vi "Forebrain.vi"() -> ()   [LabVIEW 2011]
uses:
  Control 1.ctl
  MDF.ctl
  Behaviour.ctl
  Position.ctl
  WhereAmI.ctl
  ForebrainCmd.ctl
  <vilib>/userdefined/High Color/IMAQdx.ctl
  <vilib>/vision/Image Controls.llb/IMAQ Image.ctl
  OccGrid.ctl
  Behavior.vi
  <vilib>/vision/driver/NI_Vision_Acquisition_Software.lvlib
  <vilib>/vision/NI_Vision_Development_Module.lvlib
panel:
  in  "stop":bool
  out "Draw?":bool
  in  "Tab Control":T1(tab)
  in  "CompletedMDF":bool
  in  "ResetWaypoints":bool
  in  "Behaviour":T2
  out "No. of Waypoints":i16
  out "Waypoint Index":i16
  in  "Speed":dbl(slide) scale=0.0..10.0
  out "Mission Definition":T3
  out "Mission Def File":T4[](array[typedef])
  out "Occupancy Grid 2":T5(plugin-control)
  out "Behavior":string
  in  "Camera Name":T6
  out "Occupancy Grid":T5(plugin-control)
  out "x":sgl[](array[numeric])
  out "y":sgl[](array[numeric])
  out "OccupancyGrid (Raw Data)":i8[][](array[numeric])
  out "Working":bool
  in  "stop 2":bool
  out "Dock 2":cluster{"x":sgl, "y":sgl}
  out "Bouy 1":cluster{"x":sgl, "y":sgl}
  out "Boat 2":T7
  out "Nothing":cluster{"x":sgl, "y":sgl}
  out "Working Image":T5(plugin-control)
  in  "Camera/File?":bool
  in  "Image file name":string="real pool targets rotated.bmp"
  out "Wall Position 1":T4
  out "FB Act Command":dbl[](graph)
  out "Image":T5(plugin-control)
  out "Buoy2":T8
  out "Buoy1":T8
  out "Dock":T8
  out "Real-Time MDF":T4[](array[typedef])
  out "Boat":T7
  out "Current State":i32
  out "AutoModeStop":bool
  out "Forebrain Command":T9
  out "Alive?":bool
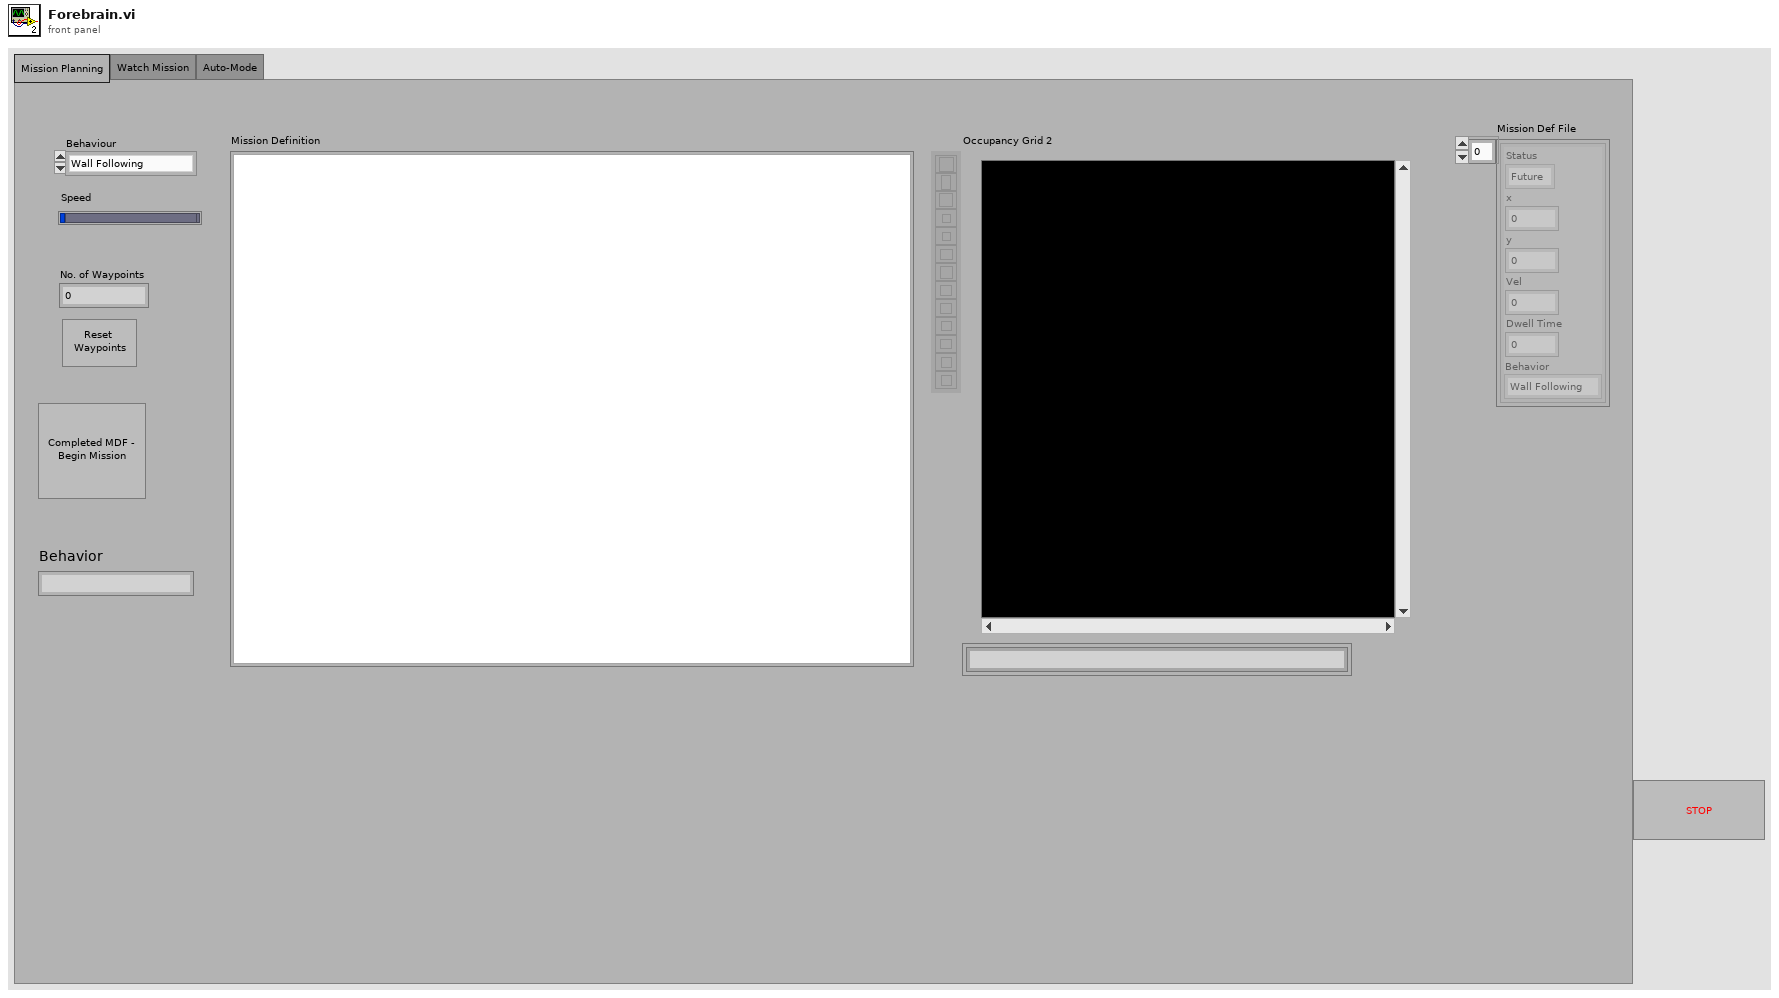
[diagram p1: front panel]
types:
  T1 = enum32{"Mission Planning", "Watch Mission", "Auto-Mode"}
  T2 = typedef "Behaviour.ctl" = enum16{"Wall Following", "Open Transit", "Find Barge", "Push Barge", "Go Home"}
  T3 = typedef "Control 1.ctl" = picture
  T4 = typedef "MDF.ctl" = cluster{"Status":enum16{"Past", "Current", "Future"}, "x":dbl, "y":dbl, "Vel":dbl, "Dwell Time":dbl, "Behavior":T2}
  T5 = typedef "IMAQ Image.ctl" = refnum<image>
  T6 = typedef "IMAQdx.ctl" = refnum<k21>
  T7 = typedef "WhereAmI.ctl" = cluster{"x":sgl, "y":sgl, "Boat\nHeading":sgl}
  T8 = typedef "Position.ctl" = cluster{"X":sgl, "Y":sgl}
  T9 = typedef "ForebrainCmd.ctl" = cluster{"Velocity":dbl, "Behaviour":T2}
  T10 = typedef "Image Type" = u32
  T11 = cluster{"Status":enum16{"Past", "Current", "Future"}, "x":dbl, "y":dbl, "Vel":dbl, "Dwell Time":dbl, "Behavior":T2}[]
  T12 = cluster{"Width":u16, "Style":enum32{"Solid", "Dash", "Dot", "DashDot", "DashDotDot"}}
  T13 = cluster{"Status":enum16{"Past", "Current", "Future"}, "x":dbl, "y":dbl, "Vel":dbl, "Dwell Time":dbl, "Behaviour":T2}
  T14 = typedef "OccGrid.ctl" = i16[][]
  T15 = typedef "LVMouseTypeDef.ctl" = cluster{"Mouse Position":cluster{"X":i32, "Y":i32}, "Mouse Modifiers":cluster{"Button Down":bool, "Shift Mod":bool, "Menu Mod":bool, "Option Mod":bool}}
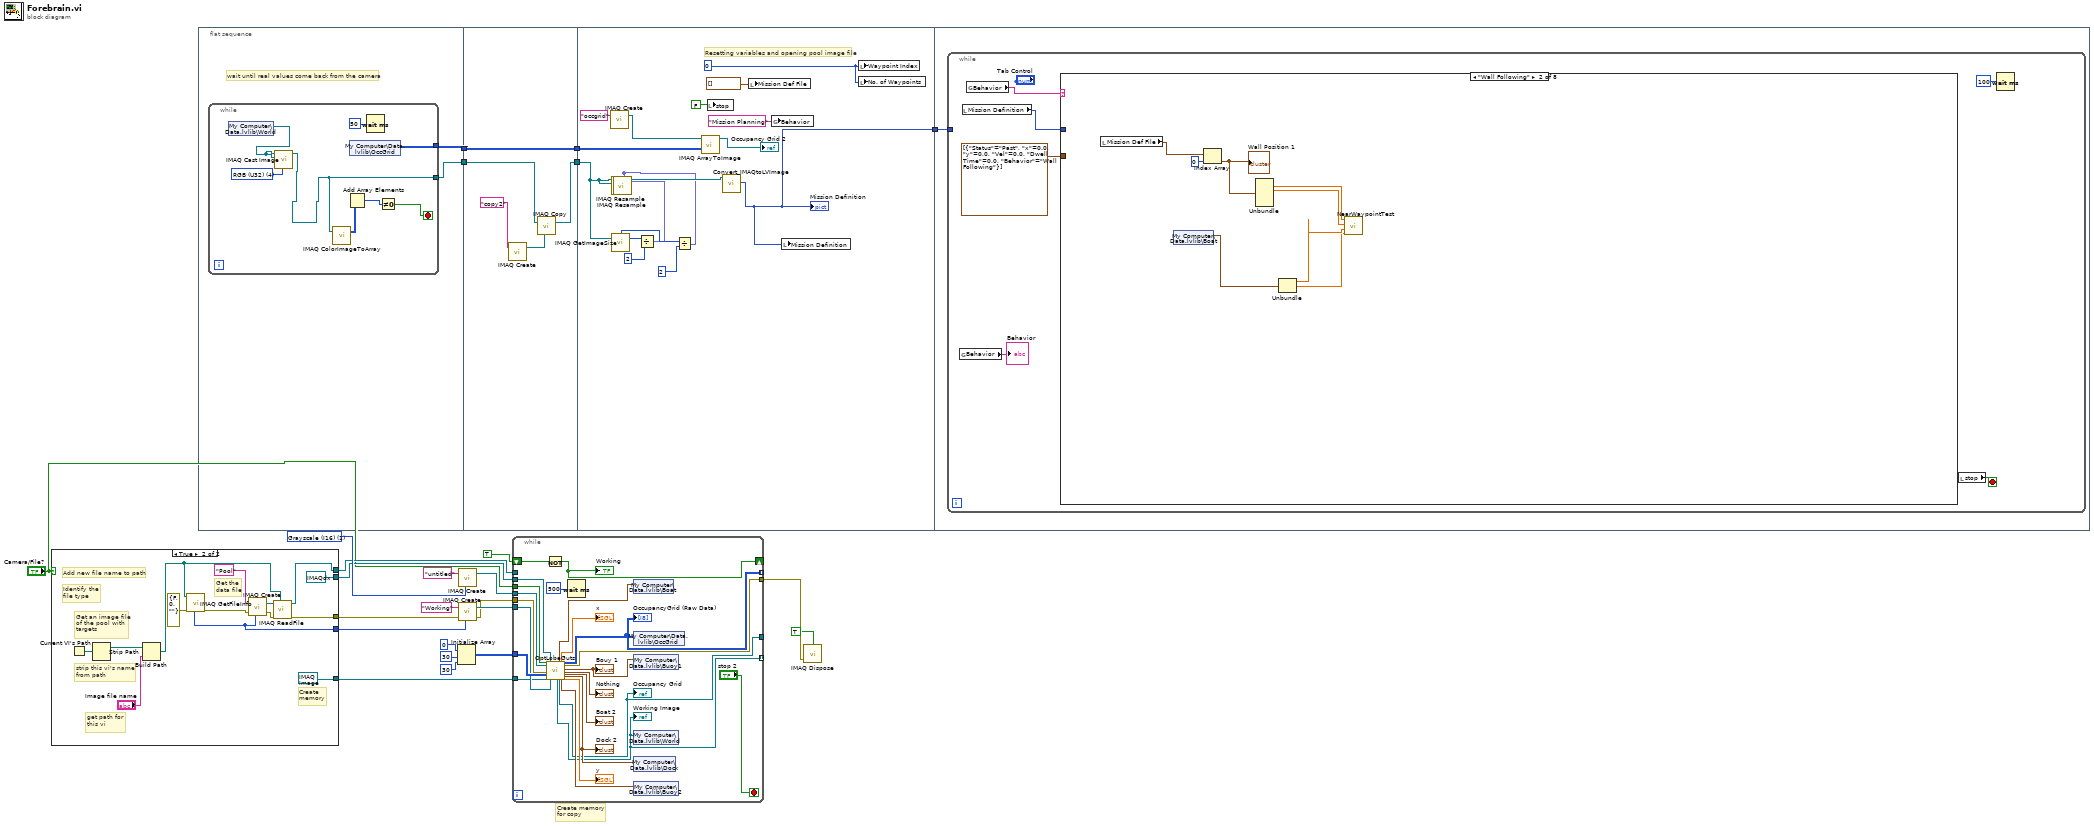
[diagram p0: block diagram]
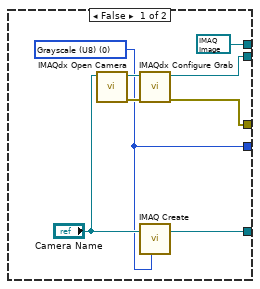
[diagram p2: hidden frame]
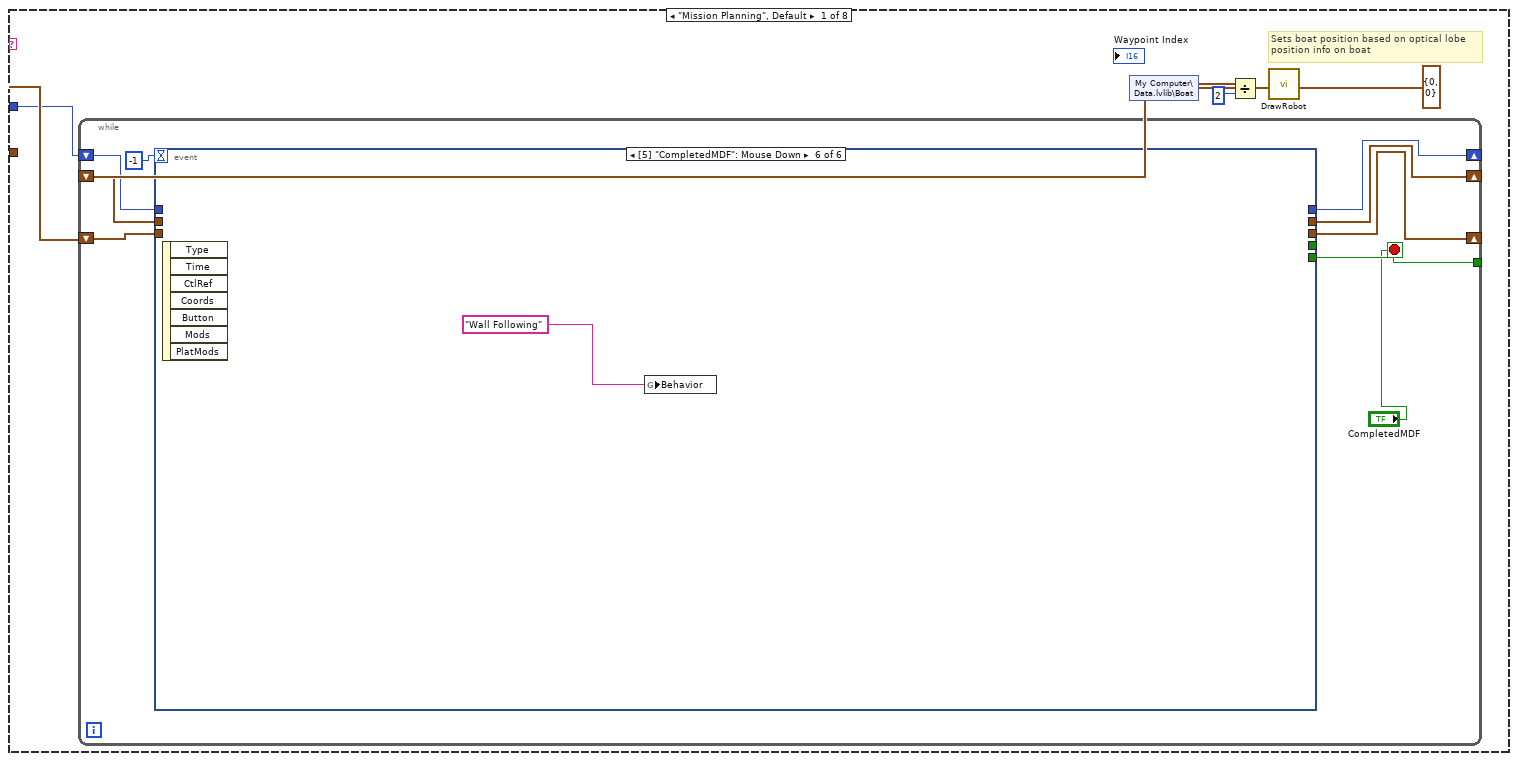
[diagram p3: hidden frame]
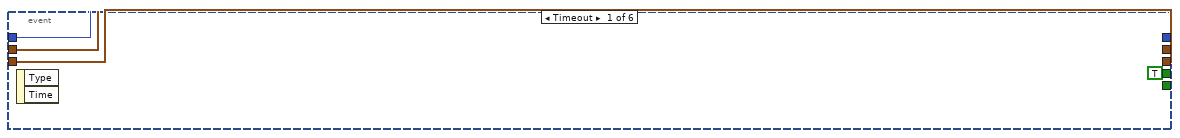
[diagram p4: hidden frame]
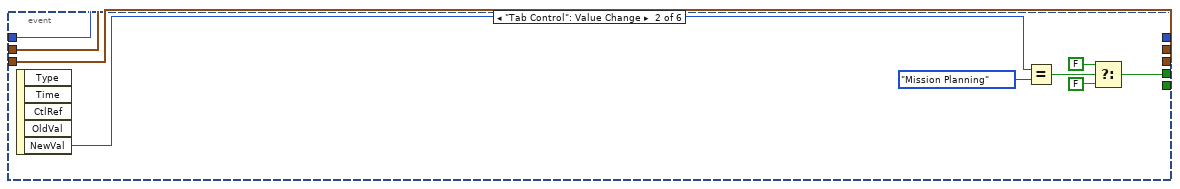
[diagram p5: hidden frame]
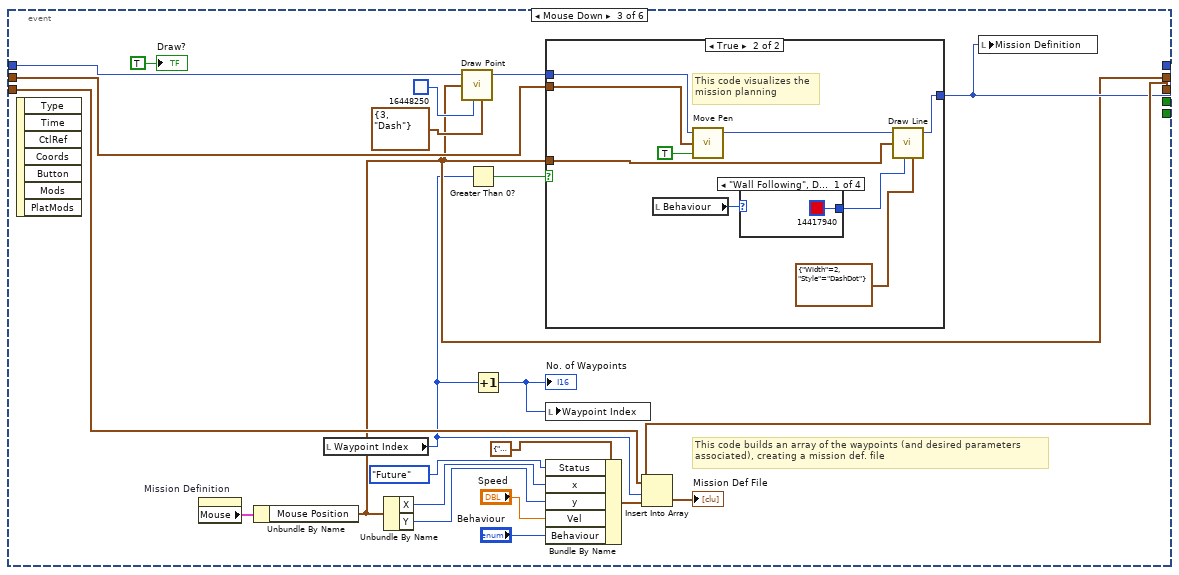
[diagram p6: hidden frame]
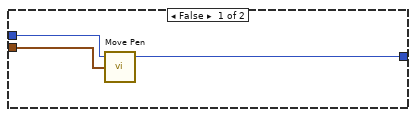
[diagram p7: hidden frame]
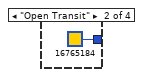
[diagram p8: hidden frame]
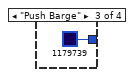
[diagram p9: hidden frame]
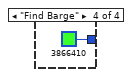
[diagram p10: hidden frame]
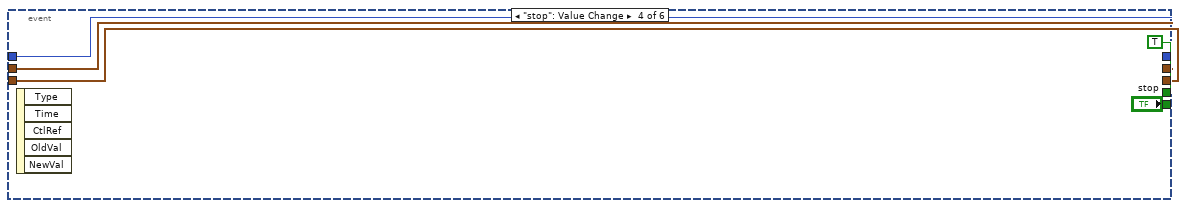
[diagram p11: hidden frame]
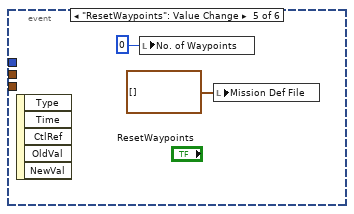
[diagram p12: hidden frame]
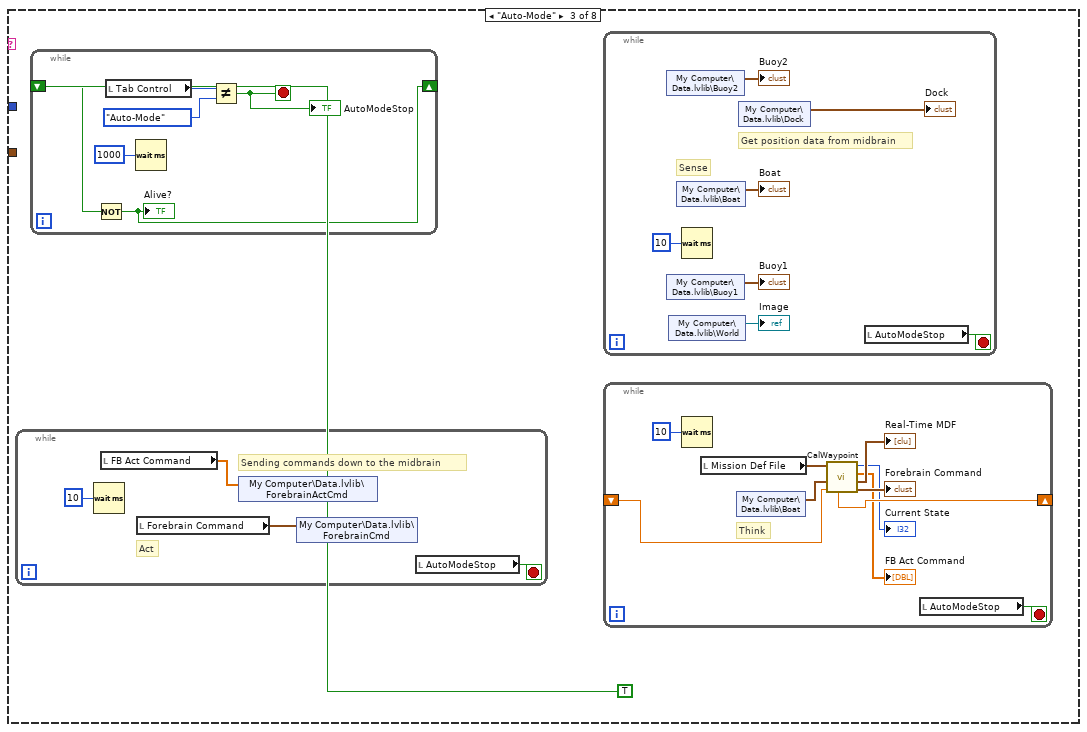
[diagram p13: hidden frame]
diagram:
  w23 = T10 1 items=["Grayscale (U8)", "Grayscale (I16)", "Grayscale (SGL)", "Complex (CSG)", "RGB (U32)", "HSL (U32)", "RGB (U64)", "Grayscale (U16)"] ("Image Type")
  # "Create memory\nfor copy"
  n1 = case shown="True" "Camera/File?" {
    tunnel: [T5 refnum ("Image Out") w37] -> w16
    tunnel: [w29 w36] -> w12
    tunnel: [w28 w35] -> w13
    tunnel: [w27 T5 refnum ("New Image")] -> w14
    tunnel: [w26 T6 refnum ("Session Out")] -> w15
    frame False {
      w28 = T10 0 items=["Grayscale (U8)", "Grayscale (I16)", "Grayscale (SGL)", "Complex (CSG)", "RGB (U32)", "HSL (U32)", "RGB (U64)", "Grayscale (U16)"] ("Image Type")
      n2 = call <vilib>:"IMAQdx Open Camera.vi"("Session In"="Camera Name") -> ("error out"=w32:errorcluster, "Session Out"=w31:T6)  [unwired: 2 in, 7 out]
      n3 = call <vilib>:"IMAQdx Configure Grab.vi"("error in"=w32, "Session In"=w31) -> ("error out"=w29:errorcluster, "Session Out"=w26:T6)  [unwired: 8 out]
      n4 = call "IMAQ Create"("Image Name"="Camera Name", "Image Type"=w28) -> ("New Image"=w27:T5)  [unwired: 2 in, 2 out]
    }
    frame True {
      # "Add new file name to path"
      # "strip this vi's name \nfrom path"
      # "get path for \nthis vi"
      # "Get the \ndata file"
      # "Create \nmemory"
      # "Identify the \nfile type"
      # "Get an image file\nof the pool with\ntargets"
      n5 = Current VI's Path() -> (path=w40:path)
      n6 = Strip Path(path=w40) -> (stripped path=w39:path)  [unwired: 1 out]
      n7 = Build Path(base path=w39, name or relative path="Image file name") -> (appended path=w38:path)
      n8 = call "IMAQ GetFileInfo"("error in (no error)"=errorcluster {"status"=FALSE, "code"=0, "source"=""}, "File Path"=w38) -> ("error out"=w46:errorcluster, "Image Type"=w35:T10)  [unwired: 3 in, 5 out]
      n9 = call "IMAQ Create"("Image Name"="Pool", "Image Type"=w35, "error in (no error)"=w46) -> ("New Image"=w44:T5, "error out"=w42:errorcluster)  [unwired: 2 in]
      n10 = call "IMAQ ReadFile"("File Path"=w38, "error in (no error)"=w42, "Image"=w44) -> ("error out"=w36:errorcluster, "Image Out"=w37:T5)  [unwired: 4 in, 3 out]
    }
  }
  n11 = flat-sequence {
    tunnel: [w48] -> w7
    tunnel: [w47] -> w5
    tunnel: w7 -> [w61]
    tunnel: [w61] -> w6
    tunnel: w5 -> [w59]
    tunnel: [w58] -> w4
    tunnel: w6 -> [w73]
    tunnel: w4 -> [w63]
    tunnel: [w62] -> w1
    tunnel: w1 -> [w79]
    frame #0 {
      # "wait until real values come back from the camera"
      n12 = while {
        tunnel: [w54] -> w48
        tunnel: [w49] -> w47
        stop <- w55 stop-if-true
        w52 = T10 4 items=["Grayscale (U8)", "Grayscale (I16)", "Grayscale (SGL)", "Complex (CSG)", "RGB (U32)", "HSL (U32)", "RGB (U64)", "Grayscale (U16)"] ("Image Type")
        n13 = shared-variable "My Computer\\Data.lvlib\\World"() -> (w53:refnum<image>)  [unwired: 1 in, 1 out]
        n14 = call "IMAQ Cast Image"("Image Type"=w52, "Image Dst"=w53, "Image Src"=w53) -> ("Image Dst Out"=w49:T5)  [unwired: 7 in, 1 out]
        n15 = call "IMAQ ColorImageToArray"("Image"=w49) -> ("Image Pixels (U32)"=w51:u32[][])  [unwired: 3 in, 2 out]
        n16 = Add Array Elements(numeric array=w51) -> (sum=w56:u32)
        n17 = shared-variable "My Computer\\Data.lvlib\\OccGrid"() -> (w54:T14)  [unwired: 1 in, 1 out]
        n18 = Wait (ms)(milliseconds to wait=u32 50) -> ()  [unwired: 1 out]
        n19 = Not Equal To 0?(x=w56) -> (x != 0?=w55:bool)
      }
    }
    frame #1 {
      n20 = call "IMAQ Create"("Image Name"="copy2") -> ("New Image"=w60:T5)  [unwired: 4 in, 1 out]
      n21 = call "IMAQ Copy"("Image Dst"=w60, "Image Src"=w59) -> ("Image Dst Out"=w58:T5)  [unwired: 4 in, 1 out]
    }
    frame #2 {
      w78 = i16 0 ("No. of Waypoints")
      # "Resetting variables and opening pool image file"
      n22 = call "IMAQ Create"("Image Name"="occgrid") -> ("New Image"=w71:T5)  [unwired: 4 in, 1 out]
      n23 = call "IMAQ GetImageSize"("Image"=w63) -> ("Y Resolution"=w70:i32, "X Resolution"=w67:i32)  [unwired: 3 in, 1 out]
      n24 = Divide(x=w70, y=2) -> (x/y=w65:fxp<+/-,32,32>)
      n25 = Divide(x=w67, y=2) -> (x/y=w64:fxp<+/-,32,32>)
      n26 = call "IMAQ Resample"("X Resolution"=w64, "Y Resolution"=w65, "Image Dst"=w63, "Image Src"=w63) -> ("Image Dst Out"=w66:T5)  [unwired: 6 in, 1 out]
      n27 = call "IMAQ Resample"("X Resolution"=w64, "Y Resolution"=w65, "Image Src"=w63) -> ()  [unwired: 7 in, 2 out]
      n28 = call "IMAQ ArrayToImage"("Image Pixels (I16)"=w73, "Image"=w71) -> ("Image Out"=→"Occupancy Grid 2":T5)  [unwired: 8 in, 1 out]
      n29 = local write "stop"(FALSE ("stop")) -> ()
      n30 = call "Convert_IMAQtoLVImage.vi"("IMAQImage In (RGB 32)"=w66) -> ("Image 2D"=w62:picture)  [unwired: 7 in, 3 out]
      "Mission Definition" <- w62
      n31 = local write "Mission Def File"(T11 [] ("MDF")) -> ()
      n32 = global write "Behavior.vi" "Behavior"("Mission Planning" ("Behavior")) -> ()
      n33 = local write "Mission Definition"(w62) -> ()
      n34 = local write "Waypoint Index"(w78) -> ()
      n35 = local write "No. of Waypoints"(w78) -> ()
    }
    frame #3 {
      n36 = while {
        tunnel: w79 -> [_]
        stop <- w84 stop-if-true
        n37 = global read "Behavior.vi" "Behavior"() -> (→"Behavior":string)
        n38 = local read "Mission Definition"() -> (w80:T3)
        n39 = global read "Behavior.vi" "Behavior"() -> (w83:string)
        n40 = case shown="\"Wall Following\"" w83 {
          tunnel: T4[] [{"Status"=enum."Past", "x"=0.0, "y"=0.0, "Vel"=0.0, "Dwell Time"=0.0, "Behavior"=enum."Wall Following"}] ("MDF") -> [w91 _ _ _ _ _ _ _]
          tunnel: w80 -> [w86 _ _ _ _ _ _ _]
          frame "Mission Planning", Default {
            # "Sets boat position based on optical lobe\nposition info on boat"
            n41 = while {
              shift-right: [w97] -> _
              shift-left: w91 -> [w100]
              shift-right: [w98] -> _
              shift-left: w86 -> [w99]
              shift-right: [w96] -> _
              shift-left: cluster{"X":i32, "Y":i32} {"X"=0, "Y"=0} ("Mouse Position") -> [w95]
              tunnel: [w94] -> _
              stop <- "CompletedMDF" stop-if-true
              n42 = event shown="[5] \"CompletedMDF\": Mouse Down" {
                selector: _ -> [_ _ _ _ _ _]
                dyn-events: _ -> [_ _ _ _ _ _]
                timeout: -1 -> [_ _ _ _ _ _]
                tunnel: w100 -> [w104 w108 w124 w152 _ _]
                tunnel: [w104 w108 w125 w152 _ _] -> w97
                tunnel: [TRUE ("t") w107 _ TRUE ("t") _ _] -> _
                tunnel: w99 -> [w102 w105 w122 w153 _ _]
                tunnel: [w102 w105 w118 w153 _ _] -> w98
                tunnel: [w103 w106 w116 w154 _ _] -> w96
                tunnel: w95 -> [w103 w106 w120 w154 _ _]
                tunnel: [_ _ _ "stop" _ _] -> w94
                event Timeout {
                  n43 = event-data() -> ()  [unwired: 1 in, 2 out]
                }
                event "Tab Control": Value Change {
                  n44 = event-data() -> ("NewVal"=w113:T1)  [unwired: 1 in, 4 out]
                  n45 = Equal?(x=w113, y=enum32{"Mission Planning", "Auto-Mode"}."Mission Planning") -> (x = y?=w111:bool)
                  n46 = Select(t=FALSE, s=w111, f=FALSE) -> (s? t:f=w107:bool)
                }
                event Mouse Down {
                  # "This code builds an array of the waypoints (and desired parameters\nassociated), creating a mission def. file"
                  n47 = event-data() -> ()  [unwired: 1 in, 7 out]
                  n48 = property on="Mission Definition" class="Pict"() -> ("Mouse"=w114:T15)  [unwired: 2 in, 2 out]
                  n49 = Unbundle By Name(w114) -> ("Mouse Position"=w116:cluster{"X":i32, "Y":i32})
                  n50 = local read "Waypoint Index"() -> (w115:i16)
                  n51 = Unbundle By Name(w116) -> ("X"=w134:i32, "Y"=w133:i32)
                  n52 = call <vilib>:"Draw Point.vi"("picture"=w122, "point(x,y)"=w116, "color(black)"=u32 16448250, "pen"=T12 {"Width"=3, "Style"=enum."Dash"}) -> ("new picture"=w119:picture)  [unwired: 5 in]
                  n53 = Greater Than 0?(x=w115) -> (x > 0?=w123:bool)
                  n54 = Increment(x=w115) -> (x+1=w132:i16)
                  "No. of Waypoints" <- w132
                  n55 = case shown="True" w123 {
                    tunnel: w116 -> [_ w145]
                    tunnel: [w136 w144] -> w118
                    tunnel: w120 -> [w135 w143]
                    tunnel: w119 -> [w137 w140]
                    frame False {
                      n56 = call <vilib>:"Move Pen.vi"("new position"=w135, "picture"=w137) -> ("new picture"=w136:picture)  [unwired: 3 in]
                    }
                    frame True {
                      # "This code visualizes the\nmission planning"
                      n57 = local read "Behaviour"() -> (w142:T2)
                      n58 = call <vilib>:"Move Pen.vi"("absolute coordinates?(T)"=TRUE, "new position"=w143, "picture"=w140) -> ("new picture"=w139:picture)  [unwired: 2 in]
                      n59 = case shown="\"Wall Following\", Default" w142 {
                        tunnel: [u32 14417940 ("color(black)") u32 16765184 ("color(black)") u32 1179739 ("color(black)") u32 3866410 ("color(black)")] -> w141
                        frame "Wall Following", Default {
                        }
                        frame "Open Transit" {
                        }
                        frame "Push Barge" {
                        }
                        frame "Find Barge" {
                        }
                      }
                      n60 = call <vilib>:"Draw Line.vi"("picture"=w139, "end point"=w145, "color(black)"=w141, "pen"=T12 {"Width"=2, "Style"=enum."DashDot"}) -> ("new picture"=w144:picture)  [unwired: 5 in]
                    }
                  }
                  n61 = local write "Waypoint Index"(w132) -> ()
                  n62 = Bundle By Name(cluster=T13 {"Status"=enum."Future", "x"=0.0, "y"=0.0, "Vel"=0.0, "Dwell Time"=0.0, "Behaviour"=enum."Wall Following"} ("MissionDefinitionFile"), "Status"=enum16{"Past", "Current", "Future"}."Future", "x"=w134, "y"=w133, "Vel"="Speed", "Behaviour"="Behaviour") -> (w127:T13)
                  n63 = Insert Into Array(array=w124, index=w115, new element=w127) -> (w125:T4[])
                  "Mission Def File" <- w125
                  n64 = local write "Mission Definition"(w118) -> ()
                  "Draw?" <- TRUE ("Draw?")
                }
                event "stop": Value Change {
                  n65 = event-data() -> ()  [unwired: 1 in, 5 out]
                }
                event "ResetWaypoints": Value Change {
                  n66 = event-data() -> ()  [unwired: 1 in, 5 out]
                  n67 = local write "No. of Waypoints"(i16 0 ("No. of Waypoints")) -> ()
                  n68 = local write "Mission Def File"(T4[] [] ("Mission Def File")) -> ()
                }
                event "CompletedMDF": Mouse Down {
                  n69 = event-data() -> ()  [unwired: 1 in, 7 out]
                  n70 = global write "Behavior.vi" "Behavior"("Wall Following" ("Behavior")) -> ()
                }
              }
            }
            n71 = shared-variable "My Computer\\Data.lvlib\\Boat"() -> (w89:T7)  [unwired: 1 in, 1 out]
            n72 = Divide(x=w89, y=2) -> (x/y=w88:T7)
            n73 = call "DrawRobot.vi"("Boat (New)"=w88) -> ()  [unwired: 9 in, 1 out]
          }
          frame "Wall Following" {
            n74 = local read "Mission Def File"() -> (w166:T4[])
            n75 = shared-variable "My Computer\\Data.lvlib\\Boat"() -> (w164:T7)  [unwired: 1 in, 1 out]
            n76 = Index Array(array=w166, index=0) -> (element=w161:T4)
            "Wall Position 1" <- w161
            n77 = Unbundle(w161) -> ("x"=w160:dbl, "y"=w159:dbl)  [unwired: 4 out]
            n78 = Unbundle(w164) -> ("x"=w163:sgl, "y"=w162:sgl)  [unwired: 1 out]
            n79 = call "NearWaypointTest.vi"("Yrobot"=w162, "Xrobot"=w163, "Ywaypoint"=w159, "Xwaypoiny"=w160) -> ()  [unwired: 7 in, 1 out]
          }
          frame "Auto-Mode" {
            n80 = while {
              stop <- w177 stop-if-true
              # "Sending commands down to the midbrain"
              # "Act"
              n81 = Wait (ms)(milliseconds to wait=u32 10) -> ()  [unwired: 1 out]
              n82 = local read "FB Act Command"() -> (w174:dbl[])
              n83 = local read "Forebrain Command"() -> (w176:T9)
              n84 = shared-variable "My Computer\\Data.lvlib\\ForebrainActCmd"(w174) -> ()  [unwired: 1 in, 1 out]
              n85 = shared-variable "My Computer\\Data.lvlib\\ForebrainCmd"(w176) -> ()  [unwired: 1 in, 1 out]
              n86 = local read "AutoModeStop"() -> (w177:bool)
            }
            n87 = while {
              shift-right: [w168] -> _
              shift-left: TRUE -> [w169]
              stop <- w171 stop-if-true
              n88 = Not(x=w169) -> (.not. x?=w168:bool)
              "Alive?" <- w168
              n89 = local read "Tab Control"() -> (w173:T1)
              n90 = Wait (ms)(milliseconds to wait=u32 1000) -> ()  [unwired: 1 out]
              n91 = Not Equal?(x=w173, y=enum32{"Mission Planning", "Auto-Mode"}."Auto-Mode") -> (x != y?=w171:bool)
              "AutoModeStop" <- w171
            }
            n92 = while {
              stop <- w188 stop-if-true
              # "Get position data from midbrain"
              # "Sense"
              n93 = shared-variable "My Computer\\Data.lvlib\\Buoy2"() -> (→"Buoy2":T8)  [unwired: 1 in, 1 out]
              n94 = shared-variable "My Computer\\Data.lvlib\\Buoy1"() -> (→"Buoy1":T8)  [unwired: 1 in, 1 out]
              n95 = shared-variable "My Computer\\Data.lvlib\\World"() -> (→"Image":refnum<image>)  [unwired: 1 in, 1 out]
              n96 = shared-variable "My Computer\\Data.lvlib\\Boat"() -> (→"Boat":T7)  [unwired: 1 in, 1 out]
              n97 = Wait (ms)(milliseconds to wait=u32 10) -> ()  [unwired: 1 out]
              n98 = shared-variable "My Computer\\Data.lvlib\\Dock"() -> (→"Dock":T8)  [unwired: 1 in, 1 out]
              n99 = local read "AutoModeStop"() -> (w188:bool)
            }
            n100 = while {
              shift-right: [w183] -> _
              shift-left: _ -> [w182]
              stop <- w187 stop-if-true
              # "Think"
              n101 = Wait (ms)(milliseconds to wait=u32 10) -> ()  [unwired: 1 out]
              n102 = local read "Mission Def File"() -> (w186:T4[])
              n103 = shared-variable "My Computer\\Data.lvlib\\Boat"() -> (w184:T7)  [unwired: 1 in, 1 out]
              n104 = call "CalWaypoint.vi"("CurrentSteerAngle"=w182, "WhereAmI?"=w184, "MDD In"=w186) -> ("Forebrain Command"=→"Forebrain Command":T9, "MDF Out"=→"Real-Time MDF":T4[], "ActCommand"=→"FB Act Command":dbl[], "Current State"=→"Current State":i32, "SteerAngle"=w183:dbl)  [unwired: 2 in, 2 out]
              n105 = local read "AutoModeStop"() -> (w187:bool)
            }
          }
          frame "Waypoint" {
          }
          frame "Find Barge" {
          }
          frame "Ram Barge" {
          }
          frame "Go Home" {
          }
          frame "Return Home" {
          }
        }
        n106 = local read "stop"() -> (w84:bool)
        n107 = Wait (ms)(milliseconds to wait=u32 100) -> ()  [unwired: 1 out]
      }
    }
  }
  n108 = Initialize Array(i16 0 ("element"), 30 ("dimension size"), 30 ("dimension size")) -> (w21:i16[][])
  n109 = call "IMAQ Create"("Image Name"="untitled", "Image Type"=w23) -> ("New Image"=w22:T5)  [unwired: 3 in, 1 out]
  n110 = call "IMAQ Create"("Image Name"="Working", "Image Type"=w13, "error in (no error)"=w12) -> ("New Image"=w11:T5, "error out"=w9:errorcluster)  [unwired: 2 in]
  n111 = while {
    tunnel: w9 -> [w212]
    tunnel: w11 -> [w200]
    tunnel: [w210] -> w3
    tunnel: w14 -> [w199]
    tunnel: w15 -> [w211]
    tunnel: w16 -> [_]
    tunnel: "Camera/File?" -> [w214]
    shift-right: [w215] -> _
    shift-left: TRUE -> [w216]
    tunnel: w21 -> [w213]
    tunnel: w22 -> [w202]
    tunnel: [w198] -> _ mode=indexing
    tunnel: [w197] -> _ mode=indexing
    tunnel: [w196] -> _
    stop <- "stop 2" stop-if-true
    n112 = Not(x=w216) -> (.not. x?=w215:bool)
    "Working" <- w215
    n113 = call "OptLobeGuts.vi"("Boolean"=w214, "source"=w202, "error in (no error)"=w212, "Array"=w213, "New Image"=w199, "Session Out"=w211, "Image Dst"=w200) -> ("Working Image"=w198:T5, 16:"Boat"=w209:T7, "Occupancy Grid"=w196:T5, "x"=→"x":sgl[], "Buoy 2"=w201:cluster{"x":sgl, "y":sgl}, "OccupancyGrid (Raw Data)"=w197:i8[][], "error out"=w210:errorcluster, "Bouy 1"=w203:cluster{"x":sgl, "y":sgl}, "Nothing"=→"Nothing":cluster{"x":sgl, "y":sgl}, 25:"Boat"=→"Boat 2":T7, "Dock"=w204:cluster{"x":sgl, "y":sgl}, "y"=→"y":sgl[])  [unwired: 8 in, 1 out]
    "Working Image" <- w198
    "Bouy 1" <- w203
    "Dock 2" <- w204
    "OccupancyGrid (Raw Data)" <- w197
    "Occupancy Grid" <- w196
    n114 = Wait (ms)(milliseconds to wait=u32 500) -> ()  [unwired: 1 out]
    n115 = shared-variable "My Computer\\Data.lvlib\\Boat"(w209) -> ()  [unwired: 1 in, 1 out]
    n116 = shared-variable "My Computer\\Data.lvlib\\OccGrid"(w197) -> ()  [unwired: 1 in, 1 out]
    n117 = shared-variable "My Computer\\Data.lvlib\\Buoy1"(w203) -> ()  [unwired: 1 in, 1 out]
    n118 = shared-variable "My Computer\\Data.lvlib\\World"(w198) -> ()  [unwired: 1 in, 1 out]
    n119 = shared-variable "My Computer\\Data.lvlib\\Dock"(w204) -> ()  [unwired: 1 in, 1 out]
    n120 = shared-variable "My Computer\\Data.lvlib\\Buoy2"(w201) -> ()  [unwired: 1 in, 1 out]
  }
  n121 = call "IMAQ Dispose"("All Images? (No)"=TRUE, "error in (no error)"=w3) -> ()  [unwired: 4 in, 1 out]
